vi "Sonar Sensors.vi"   [LabVIEW 2011]
uses:
  jeevan/Sonar + GPS/Sonar + GPS Global Variables.vi
  <vilib>/LabVIEW Interface for Arduino/LabVIEW Interface for Arduino.lvlib
types:
  T1 = typedef "LabVIEW Interface for Arduino.lvlib/Arduino Resource.ctl" = cluster{"VISA resource":refnum<visa-resource-name>, "Board Type":T2, "Connection Type":enum8{"USB / Serial"}, "Bytes Per Packet (15)":u8}
  T2 = typedef "LabVIEW Interface for Arduino.lvlib/Board Type.ctl" = enum16{"Uno", "Dimuelanove w/Atmega 328", "Mega 2560"}
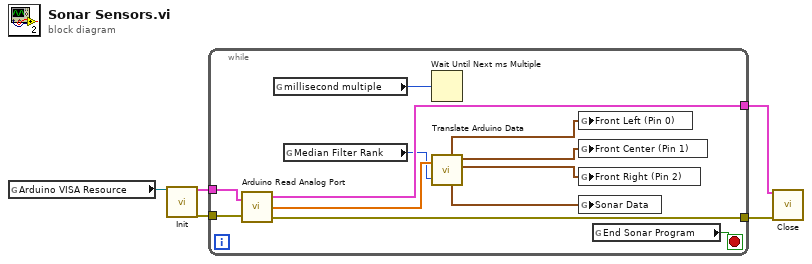
[diagram p0: block diagram]
diagram:
  n1 = global read "Sonar + GPS Global Variables.vi" "Arduino VISA Resource"() -> (w1:refnum<visa-resource-name>)
  n2 = call <vilib>:"Init.vi"("VISA resource"=w1) -> ("Arduino Resource"=w3:T1, "error out"=w2:errorcluster)  [unwired: 17 in]
  n3 = while {
    tunnel: w3 -> [w17]
    tunnel: w2 -> [w16]
    tunnel: [w15] -> w5
    tunnel: [w14] -> w4
    stop <- w6 stop-if-true
    n4 = call "Arduino Read Analog Port.vi"("Arduino Resource In"=w17, "Arduino Error In"=w16) -> ("Arduino Resource Out"=w15:T1, "Analog Port Out"=w13:dbl[], "Arduino Error Out"=w14:errorcluster)
    n5 = global read "Sonar + GPS Global Variables.vi" "millisecond multiple"() -> (w7:u32)
    n6 = global read "Sonar + GPS Global Variables.vi" "Median Filter Rank"() -> (w8:i32)
    n7 = Wait Until Next ms Multiple(millisecond multiple=w7) -> ()  [unwired: 1 out]
    n8 = call "Translate Arduino Data.vi"("Analog Port In"=w13, "Median Filter Rank"=w8) -> ("Front Left (Pin 0)"=w12:cluster{u32, u32}, "Sonar Data"=w9:cluster{dbl, dbl, dbl}, "Front Center (Pin 1)"=w11:cluster{u32, u32}, "Front Right (Pin 2)"=w10:cluster{u32, u32})  [unwired: 2 out]
    n9 = global write "Sonar + GPS Global Variables.vi" "Front Left (Pin 0)"(w12) -> ()
    n10 = global write "Sonar + GPS Global Variables.vi" "Front Center (Pin 1)"(w11) -> ()
    n11 = global write "Sonar + GPS Global Variables.vi" "Front Right (Pin 2)"(w10) -> ()
    n12 = global write "Sonar + GPS Global Variables.vi" "Sonar Data"(w9) -> ()
    n13 = global read "Sonar + GPS Global Variables.vi" "End Sonar Program"() -> (w6:bool)
  }
  n14 = call <vilib>:"Close.vi"("Arduino Resource"=w5, "error in"=w4) -> ()  [unwired: 13 in, 1 out]
